vi "ASCII 쓰기 (2D 배열저장).vi"() -> ()   [LabVIEW 2014]
uses:
  <vilib>/Analysis/NI_AALBase.lvlib
panel:
  out "스프레드시트 문자열":string
  in  "파일 경로":path
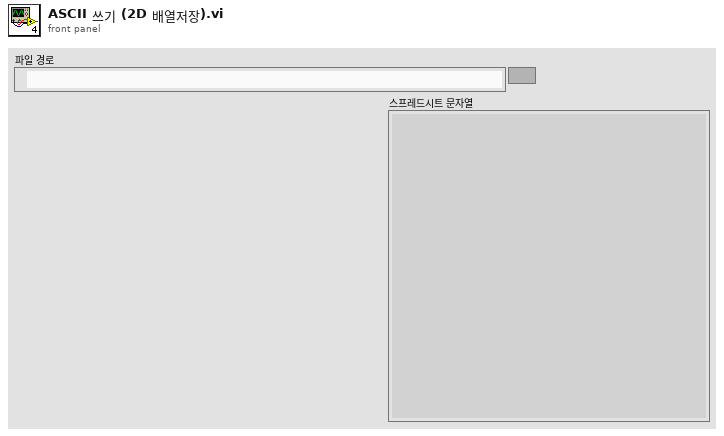
[diagram p1: front panel]
types:
  T1 = enum16{"open", "replace", "create", "open or create", "replace or create", "replace or create with confirmation"}
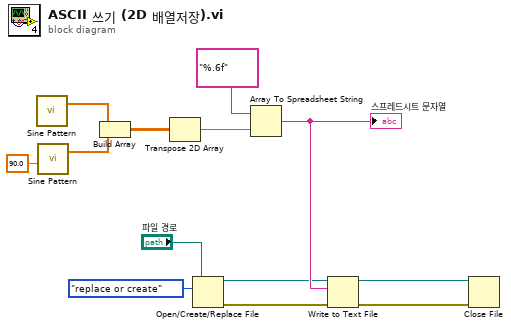
[diagram p0: block diagram]
diagram:
  n1 = call <vilib>:"Sine Pattern.vi"() -> ("Sinusoidal Pattern"=w8:dbl[])  [unwired: 4 in, 1 out]
  n2 = call <vilib>:"Sine Pattern.vi"("phase(degrees)"=90.0) -> ("Sinusoidal Pattern"=w7:dbl[])  [unwired: 3 in, 1 out]
  n3 = Build Array(w8, w7) -> (w6:dbl[][])
  n4 = Transpose 2D Array(2D array=w6) -> (transposed array=w5:dbl[][])
  n5 = Open/Create/Replace File(file path (use dialog)="파일 경로", operation (0:open)=T1."replace or create" ("동작(0:open)")) -> (refnum out=w2:refnum<file>, error out=w1:errorcluster)  [unwired: 4 in, 1 out]
  n6 = Array To Spreadsheet String(array=w5, 3:"%.6f" ("포맷 문자열")) -> (spreadsheet string=w3:string)  [unwired: 1 in]
  "스프레드시트 문자열" <- w3
  n7 = Write to Text File(file (use dialog)=w2, text=w3, error in=w1) -> (refnum out=w13:refnum<file>, error out=w12:errorcluster)  [unwired: 1 in, 1 out]
  n8 = Close File(refnum=w13, error in=w12) -> ()  [unwired: 2 out]
